vi "FindEEPROMandInputScriptPathandLetter.vi"(6 "Error In":errorcluster, 7 "Re Create New Engr Results? (F)":bool, 8 "Eng-Result #":u32, 9 "Create New Engr Results? (F)":bool) -> (0 "Error Out":errorcluster, 2 "Engr Result Path":path, 3 "Template Path":path)   [LabVIEW 2015]
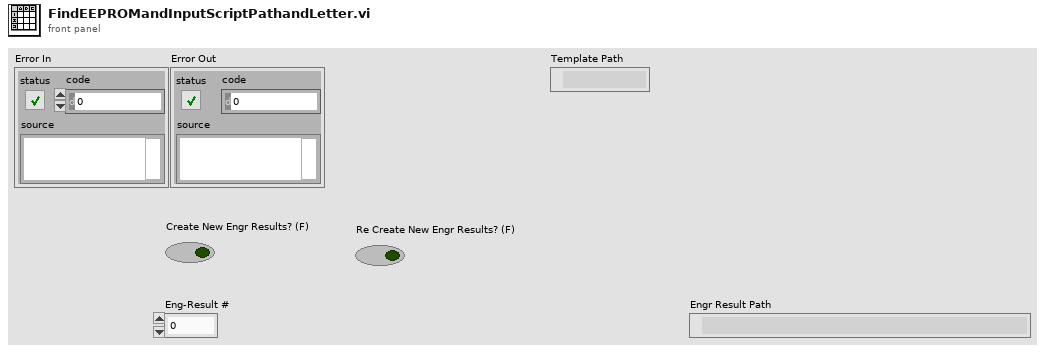
[diagram p1: front panel]
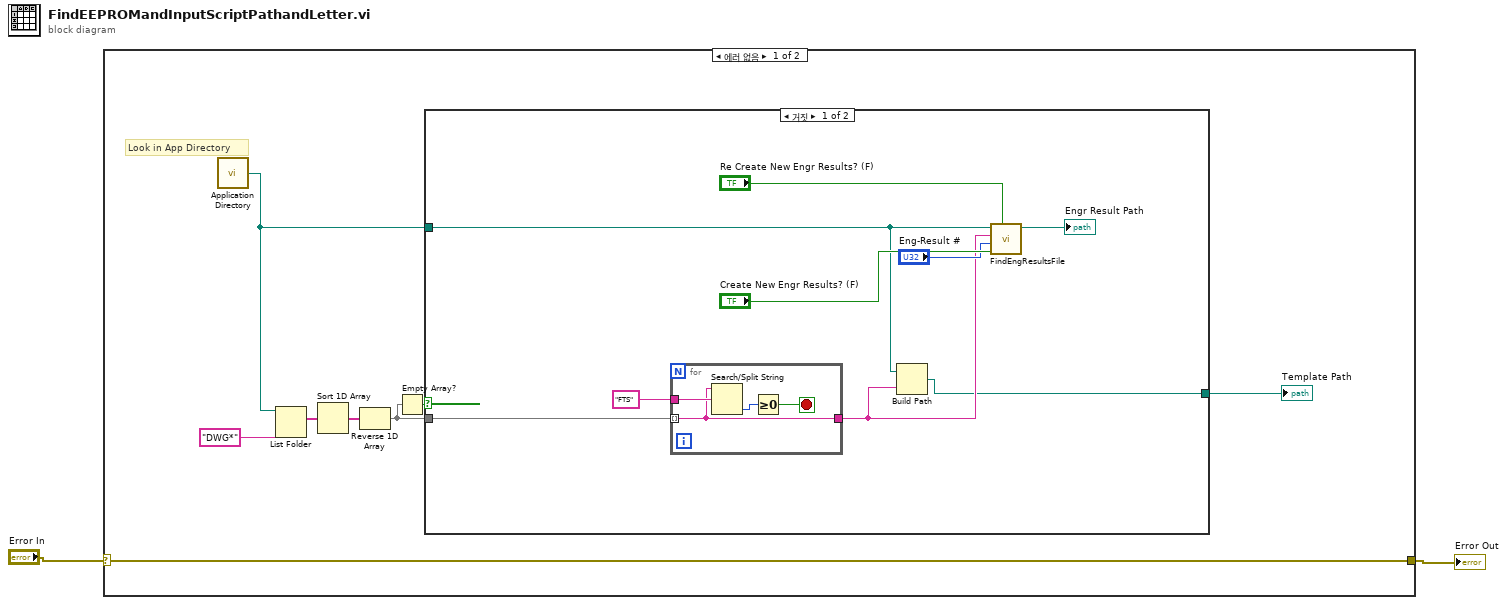
[diagram p0: block diagram]
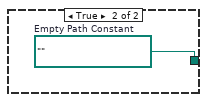
[diagram p2: hidden frame]
diagram:
  n1 = case shown="에러 없음" "Error In" {
    selector: "Error In" -> [w3 w25]
    tunnel: [w3 w25] -> w1
    frame No Error {
      # "Look in App Directory"
      n2 = call <vilib>:"Application Directory.vi"() -> ("Application Directory"=w5:path)
      n3 = List Folder(path=w5, pattern="DWG*") -> (filenames=w9:string[])  [unwired: 2 in, 3 out]
      n4 = Sort 1D Array(array=w9) -> (sorted array=w8:string[])
      n5 = Reverse 1D Array(array=w8) -> (reversed array=w6:string[])
      n6 = Empty Array?(array=w6) -> (empty?=w7:bool)
      n7 = case shown="거짓" w7 {
        tunnel: w6 -> [w19 _]
        tunnel: w5 -> [w14 _]
        tunnel: [w12 w24] -> w4
        frame False {
          n8 = for {
            tunnel: w19 -> [w21] mode=indexing
            tunnel: "FTS" -> [w23]
            tunnel: [w21] -> w13
            stop <- w20 stop-if-true
            n9 = Search/Split String(string=w21, search string/char (-)=w23) -> (offset of match=w22:i32)  [unwired: 1 in, 2 out]
            n10 = Greater Or Equal To 0?(x=w22) -> (x >= 0?=w20:bool)
          }
          n11 = Build Path(base path=w14, name or relative path=w13) -> (appended path=w12:path)
          n12 = call "FindEngResultsFile.vi"("Input Path"=w14, "EEPROM Template File"=w13, "Eng-Results"="Eng-Result #", "Create Eng Results File?"="Create New Engr Results? (F)", "Re Create Eng Results File?"="Re Create New Engr Results? (F)") -> ("Engr Result File"=→"Engr Result Path":path)  [unwired: 5 in]
        }
        frame True {
          w24 = path ""  # Empty Path Constant
        }
      }
      "Template Path" <- w4
    }
    frame Error {
    }
  }
  "Error Out" <- w1
